vi "array transformations V1.vi"(6 "phase":dbl, 7 "action":T1, 8 "array in":cdb[](array[numeric])) -> (0 "array out":cdb[](array[numeric]))   [LabVIEW 2015]
uses:
  array transformation action.ctl
panel:
  in  "Numeric Control":cdb
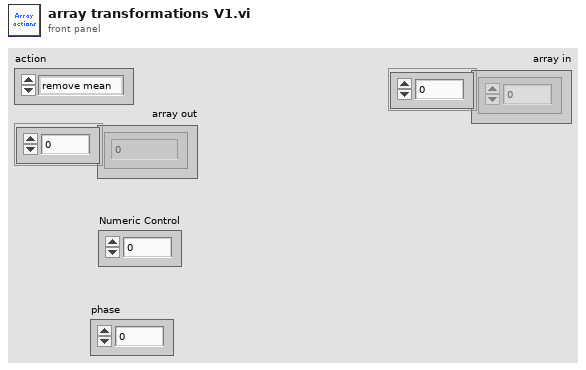
[diagram p1: front panel]
types:
  T1 = typedef "array transformation action.ctl" = enum16{"remove mean", "nomalize (by abs magn)", "rotate phase"}
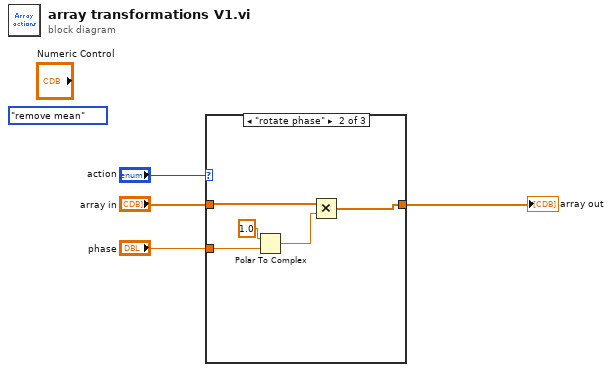
[diagram p0: block diagram]
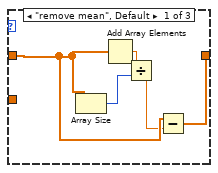
[diagram p2: hidden frame]
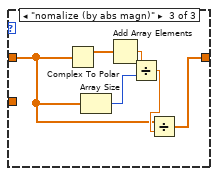
[diagram p3: hidden frame]
diagram:
  (unwired) array_transformation_action."remove mean" ("action")
  n1 = case shown="\"rotate phase\"" "action" {
    tunnel: "array in" -> [w7 w13 w16]
    tunnel: [w5 w12 w15] -> w2
    tunnel: "phase" -> [_ w11 _]
    frame "remove mean", Default {
      n2 = Array Size(array=w7) -> (size(s)=w8:i32)
      n3 = Add Array Elements(numeric array=w7) -> (sum=w9:cdb)
      n4 = Divide(x=w9, y=w8) -> (x/y=w6:cdb)
      n5 = Subtract(x=w7, y=w6) -> (x-y=w5:cdb[])
    }
    frame "rotate phase" {
      n6 = Polar To Complex(1:w11, 2:1.0 ("r")) -> (0:w14:cdb)
      n7 = Multiply(x=w13, y=w14) -> (x*y=w12:cdb[])
    }
    frame "nomalize (by abs magn)" {
      n8 = Complex To Polar(r * e^(i*theta)=w16) -> (r=w20:dbl[])  [unwired: 1 out]
      n9 = Array Size(array=w16) -> (size(s)=w18:i32)
      n10 = Add Array Elements(numeric array=w20) -> (sum=w19:dbl)
      n11 = Divide(x=w19, y=w18) -> (x/y=w17:dbl)
      n12 = Divide(x=w16, y=w17) -> (x/y=w15:cdb[])
    }
  }
  "array out" <- w2
